vi "延迟测量.vi"() -> ()   [LabVIEW 2017]
uses:
  <vilib>/Utility/file.llb/Write Delimited Spreadsheet (string).vi
panel:
  in  "step":dbl=125.0 format="%#_13g"
  out "mean[ps]":dbl=-3.0179300175540487 format="%0.2f"
  out "standard output":string="CRITICAL WARNING: [Common 17-183] Failed to open handle vivado.jou. Please check access permission of directory 'C:\\Windows\\System32'. You should restart the application from a writable working directory.\r\nCRITICAL WARNING: [Common 17-183] Failed to open handle vivado.log. Please check access permission of directory 'C:\\Windows\\System32'. You should restart the application from a writable working directory.\r\n\r\n****** Vivado v2024.1 (64-bit)\r\n  **** SW Build 5076996 on Wed May 22 18:37:14 MDT 2024\r\n  **** IP Build 5075265 on Wed May 22 21:45:21 MDT 2024\r\n  **** SharedData Build 5076995 on Wed May 22 18:29:18 MDT 2024\r\n  **** Start of session at: Sat Mar  1 13:04:09 2025\r\n    ** Copyright 1986-2022 Xilinx, Inc. All Rights Reserved.\r\n    ** Copyright 2022-2024 Advanced Micro Devices, Inc. All Rights Reserved.\r\n\r\nsource {G:\\tdc\\2017\\program_fpga.tcl}\r\n# set_part {xc7k410tffg900-3}    \r\nINFO: [Coretcl 2-1500] The part has been set to 'xc7k410tffg900-3' for the current project only. Run set_part -help for more details. To evaluate different speed grades in the current design, use the set_speed_grade command, or use the open_checkpoint -part command to change the part used by an existing checkpoint design.\r\nset_part: Time (s): cpu = 00:00:06 ; elapsed = 00:00:07 . Memory (MB): peak = 617.039 ; gain = 204.969\r\n# open_hw_manager\r\n# connect_hw_server -allow_non_jtag              \r\nINFO: [Labtools 27-2285] Connecting to hw_server url TCP:localhost:3121\r\nINFO: [Labtools 27-3415] Connecting to cs_server url TCP:localhost:0\r\nINFO: [Labtools 27-3417] Launching cs_server...\r\nINFO: [Labtools 27-2221] Launch Output:\r\n\r\n\r\n******** Xilinx cs_server v2024.1.0\r\n  ****** Build date   : Mar 09 2024-08:00:37\r\n    **** Build number : 2024.1.1709942437\r\n      ** Copyright 2017-2022 Xilinx, Inc. All Rights Reserved.\r\n      ** Copyright 2022-2025 Advanced Micro Devices, Inc. All Rights Reserved.\r\n\r\n\r\n\r\n# open_hw_target {localhost:3121/xilinx_tcf/Xilinx/0000177f546201}\r\nINFO: [Labtoolstcl 44-466] Opening hw_target localhost:3121/xilinx_tcf/Xilinx/0000177f546201\r\n# set_property PROBES.FILE {} [get_hw_devices xc7k410t_0]\r\n# set_property FULL_PROBES.FILE {} [get_hw_devices xc7k410t_0]\r\n# set_property PROGRAM.FILE {G:/fpga_tdc/FPGA/muon_TDC/top_v120_v2.bit} [get_hw_devices xc7k410t_0]\r\n# program_hw_devices [get_hw_devices xc7k410t_0]\r\nINFO: [Labtools 27-3164] End of startup status: HIGH\r\nprogram_hw_devices: Time (s): cpu = 00:00:32 ; elapsed = 00:00:33 . Memory (MB): peak = 620.281 ; gain = 0.000\r\n# close_hw_target {localhost:3121/xilinx_tcf/Xilinx/0000177f546201}\r\nINFO: [Labtoolstcl 44-464] Closing hw_target localhost:3121/xilinx_tcf/Xilinx/0000177f546201\r\n# close_hw_manager\r\n# exit\r\nINFO: [Common 17-206] Exiting Vivado at Sat Mar  1 13:04:55 2025...\r\n"
  out "error out":errorcluster
  out "ping":bool=TRUE
  out "result":string[][](array[string])=[["_20250301_010502", "42", "-1963", "31", "16"], ["_20250301_010903", "42", "-3", "28", "0"]]
  in  "data  path":path=path "G:/tdc/2017/delay.csv"
  in  "stop":bool
  in  "PMT通道B":i32=42
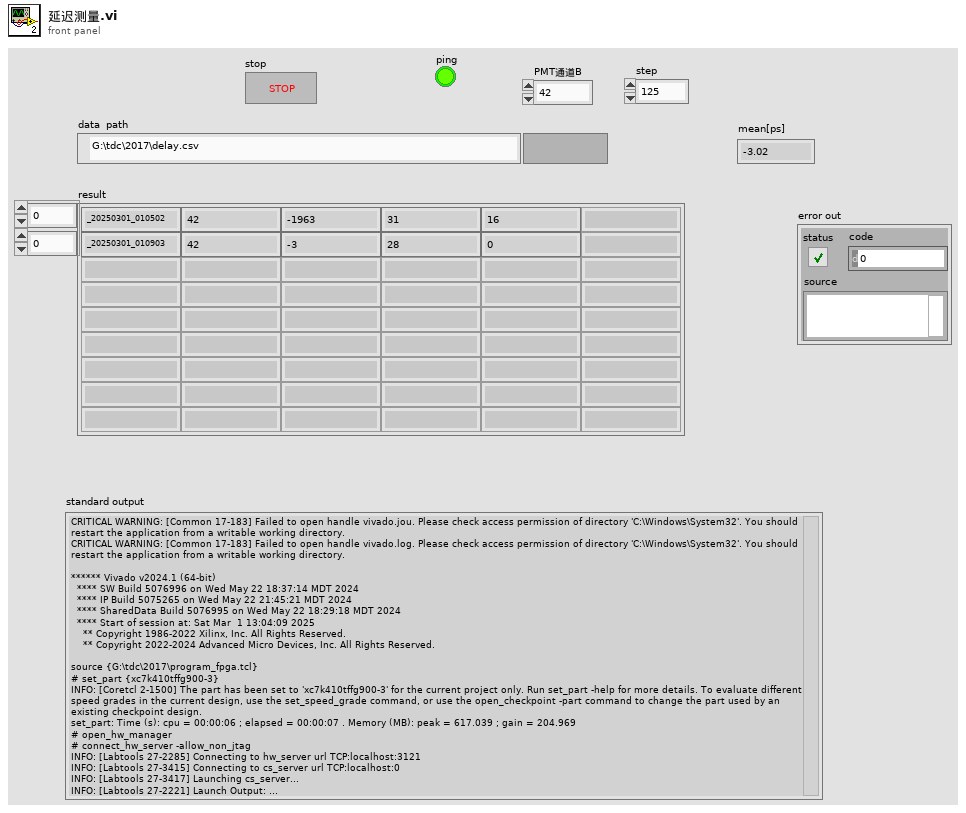
[diagram p1: front panel]
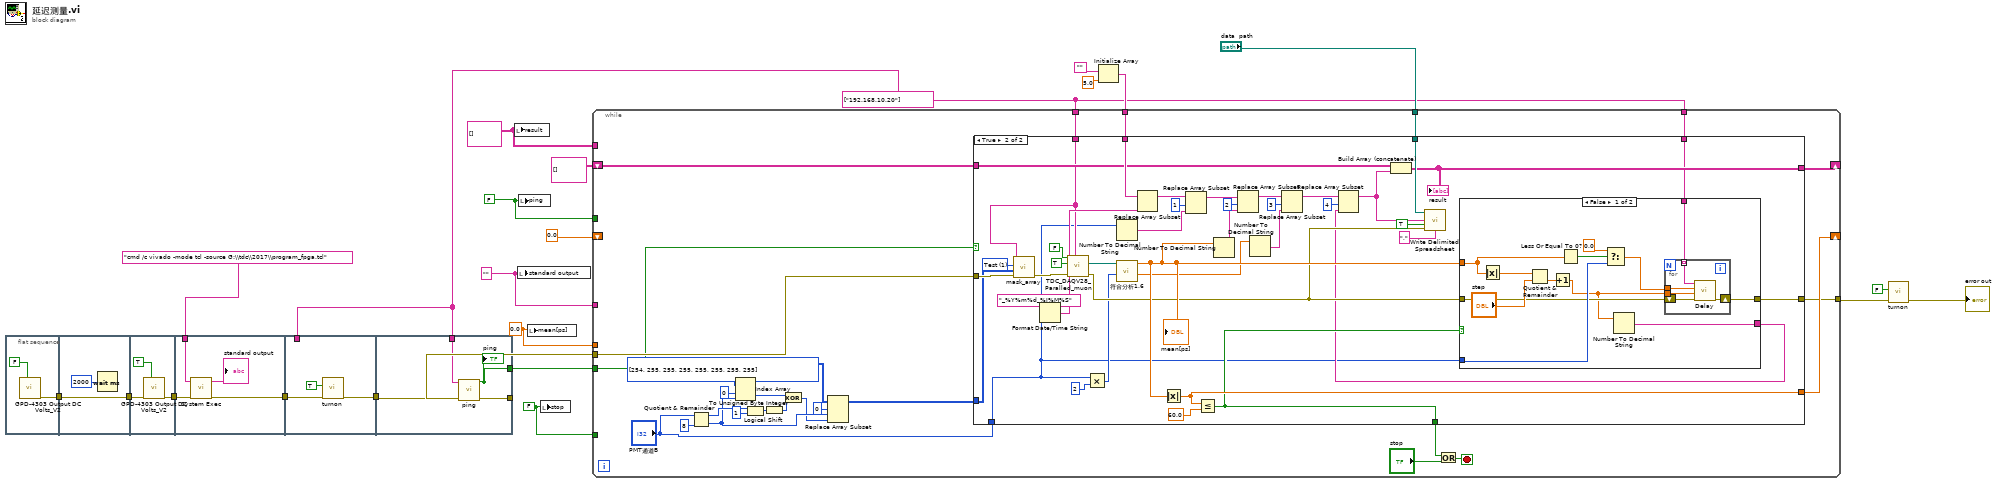
[diagram p0: block diagram]
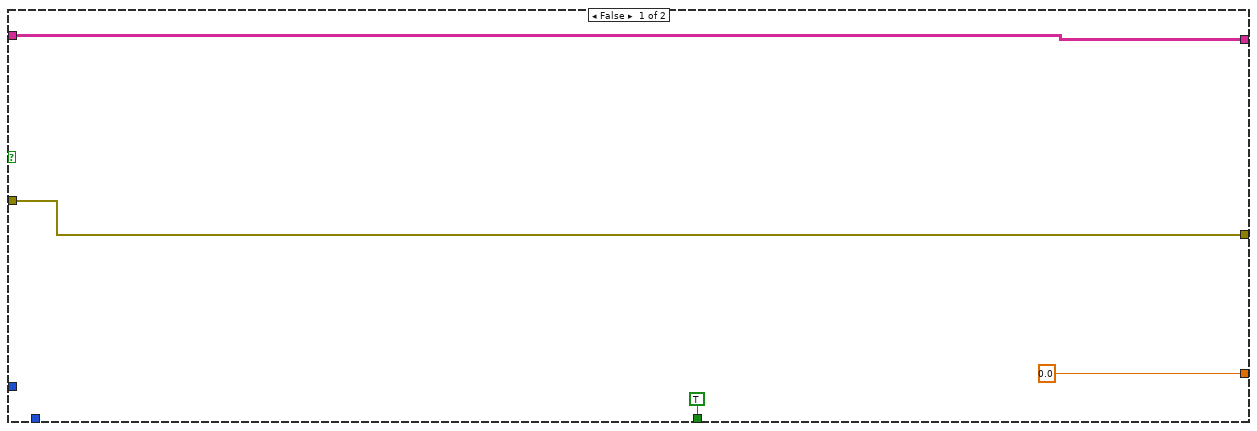
[diagram p2: hidden frame]
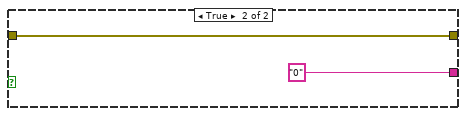
[diagram p3: hidden frame]
diagram:
  w7 = FALSE ("stop")
  w8 = 0.0 ("mean[ps]")
  w15 = "" ("standard output")
  w16 = FALSE ("ping")
  w17 = string[][] [] ("result")
  w4 = string[] ["192.168.10.20"] ("address")
  n1 = flat-sequence {
    tunnel: [w25] -> w14
    tunnel: w14 -> [w27]
    tunnel: [w27] -> w13
    tunnel: w13 -> [w29]
    tunnel: [w28] -> w12
    tunnel: w12 -> [w33]
    tunnel: "cmd /c vivado -mode tcl -source G:\\tdc\\2017\\program_fpga.tcl" ("command line") -> [w32]
    tunnel: [w34] -> w6
    tunnel: w6 -> [w37]
    tunnel: [w36] -> w5
    tunnel: w4 -> [_]
    tunnel: w5 -> [w41]
    tunnel: w4 -> [w40]
    tunnel: [w39] -> w11
    tunnel: [w38] -> w10
    frame #0 {
      n2 = call "GPD-4303 Output DC Volts_V2.vi"("Enable Output (T: Enable)"=FALSE) -> ("error out"=w25:errorcluster)  [unwired: 8 in, 2 out]
    }
    frame #1 {
      n3 = Wait (ms)(milliseconds to wait=u32 2000) -> ()  [unwired: 1 out]
    }
    frame #2 {
      n4 = call "GPD-4303 Output DC Volts_V2.vi"("Enable Output (T: Enable)"=TRUE, "error in (no error)"=w29) -> ("error out"=w28:errorcluster)  [unwired: 7 in, 2 out]
    }
    frame #3 {
      n5 = call <vilib>:"System Exec.vi"("error in (no error)"=w33, "command line"=w32) -> ("error out"=w34:errorcluster, "standard output"=→"standard output":string)  [unwired: 6 in, 2 out]
    }
    frame #4 {
      n6 = call "turnon.vi"("error in (no error)"=w37, "Enable Output (T: Enable)"=TRUE) -> ("error out"=w36:errorcluster)  [unwired: 9 in]
    }
    frame #5 {
      n7 = call "ping.vi"("error in (no error)"=w41, "address"=w40) -> ("error out"=w39:errorcluster, "ping"=w38:bool)  [unwired: 7 in, 1 out]
      "ping" <- w38
    }
  }
  n8 = local write "result"(w17) -> ()
  n9 = local write "standard output"(w15) -> ()
  n10 = local write "ping"(w16) -> ()
  n11 = local write "mean[ps]"(w8) -> ()
  n12 = local write "stop"(w7) -> ()
  n13 = Initialize Array("", 5.0 ("element")) -> (w19:string[])
  n14 = while {
    tunnel: w4 -> [w47]
    shift-right: [w65] -> _
    shift-left: 0.0 ("t") -> [_]
    tunnel: "data  path" -> [w63]
    tunnel: w19 -> [w62]
    shift-right: [w61] -> _
    shift-left: string[][] [] -> [w60]
    tunnel: [w46] -> w2
    tunnel: w17 -> [_]
    tunnel: w16 -> [_]
    tunnel: w15 -> [_]
    tunnel: w4 -> [w45]
    tunnel: w11 -> [w44]
    tunnel: w10 -> [w43]
    tunnel: w8 -> [_]
    tunnel: w7 -> [_]
    stop <- w67 stop-if-true
    w55 = u8[][] [[254, 255, 255, 255, 255, 255, 255, 255]] ("Test")
    n15 = Quotient & Remainder(x="PMT通道B", y=8) -> (x-y*floor(x/y)=w56:i32, floor(x/y)=w54:i32)
    n16 = Index Array(array=w55, index (row)=0 ("disabled index (row)"), index (col)=w54) -> (element=w52:u8)
    n17 = Logical Shift(y=w56, x=u32 1) -> (x << y=w50:u32)
    n18 = To Unsigned Byte Integer(number=w50) -> (unsigned 8bit integer=w49:u8)
    n19 = Exclusive Or(1:w49, 2:w52) -> (0:w51:u8)
    n20 = Replace Array Subset(array=w55, new element=w51, index (row)=0, index (col)=w54) -> (w48:u8[][])
    n21 = case shown="True" w43 {
      tunnel: [0.0 w107] -> w65
      tunnel: [TRUE w106] -> w64
      tunnel: w63 -> [_ w103]
      tunnel: w62 -> [_ w102]
      tunnel: [w71 w88] -> w61
      tunnel: w60 -> [w71 w87]
      tunnel: w44 -> [w70 w80]
      tunnel: w48 -> [_ w79]
      tunnel: w47 -> [_ w78]
      tunnel: [w70 w76] -> w46
      tunnel: w45 -> [_ w75]
      tunnel: "PMT通道B" -> [_ w72]
      frame False {
      }
      frame True {
        w77 = u16 1 items=["default", "Test", "NormalUse"] ("下拉列表")
        n22 = call "mask_array.vi"("error in (no error)"=w80, "Test"=w79, "下拉列表"=w77, "address"=w78) -> ("error out"=w81:errorcluster)  [unwired: 7 in]
        n23 = Format Date/Time String(time format string (%c)="_%Y%m%d_%I%M%S") -> (date/time string=w100:string)  [unwired: 2 in]
        n24 = call "TDC_DAQV28_Paralled_muon.vi"("address"=w78, "error in (no error)"=w81, "save data"=TRUE, "SMA mode"=FALSE) -> ("error out 3"=w83:errorcluster, "csv path"=w109:path)  [unwired: 5 in, 1 out]
        n25 = Multiply(x=w72, y=2) -> (x*y=w73:i32)
        n26 = Number To Decimal String(number=w72) -> (decimal integer string=w97:string)  [unwired: 1 in]
        n27 = call "符合分析1.6.vi"("通道B"=w73, "file path (dialog if empty)"=w109) -> ("Fitting Sigma"=w90:dbl, "mean[ps]"=w93:dbl)  [unwired: 5 in, 3 out]
        "mean[ps]" <- w93
        n28 = Replace Array Subset(array=w102, new element=w100) -> (w99:string[])  [unwired: 1 in]
        n29 = Absolute Value(x=w93) -> (abs(x)=w107:dbl)
        n30 = Replace Array Subset(array=w99, new element=w97, index=1) -> (w96:string[])
        n31 = Less Or Equal?(x=w107, y=60.0) -> (x <= y?=w106:bool)
        n32 = Number To Decimal String(number=w93) -> (decimal integer string=w94:string)  [unwired: 1 in]
        n33 = Replace Array Subset(array=w96, new element=w94, index=2) -> (w92:string[])
        n34 = Number To Decimal String(number=w90) -> (decimal integer string=w89:string)  [unwired: 1 in]
        n35 = Replace Array Subset(array=w92, new element=w89, index=3) -> (w86:string[])
        n36 = case shown="False" w106 {
          tunnel: w93 -> [w122 _]
          tunnel: w72 -> [w120 _]
          tunnel: w83 -> [w118 w130]
          tunnel: [w116 "0"] -> w82
          tunnel: [w115 w130] -> w76
          tunnel: w75 -> [w113 _]
          frame False {
            n37 = Absolute Value(x=w122) -> (abs(x)=w124:dbl)
            n38 = Quotient & Remainder(x=w124, y="step") -> (floor(x/y)=w117:dbl)  [unwired: 1 out]
            n39 = Increment(x=w117) -> (x+1=w112:dbl)
            n40 = Less Or Equal To 0?(x=w122) -> (x <= 0?=w114:bool)
            n41 = Select(t=0.0, s=w114, f=w120) -> (s? t:f=w119:dbl)
            n42 = Number To Decimal String(number=w112) -> (decimal integer string=w116:string)  [unwired: 1 in]
            n43 = for {
              tunnel: w119 -> [w129]
              tunnel: w112 -> [w127]
              shift-right: [w126] -> w115
              shift-left: w118 -> [w128]
              tunnel: w113 -> [w125] mode=indexing
              n44 = call "Delay.vi"("error in (no error)"=w128, "delay_value"=w127, "channel"=w129, "IP address"=w125) -> ("error out"=w126:errorcluster)  [unwired: 7 in]
            }
          }
          frame True {
          }
        }
        n45 = Replace Array Subset(array=w86, new element=w82, index=4) -> (w85:string[])
        n46 = Build Array (concatenate)(w87, w85) -> (w88:string[][])
        "result" <- w88
        n47 = call-poly <vilib>:"Write Delimited Spreadsheet.vi"("file path (dialog if empty)"=w103, "1D data"=w85, "append to file? (new file:F)"=TRUE, "error in (no error)"=w83, "delimiter (\\t)"="," ("delimiter (\\t)")) -> ()  [unwired: 9 in, 2 out]
      }
    }
    n48 = Or(x=w64, y="stop") -> (x .or. y?=w67:bool)
  }
  n49 = call "turnon.vi"("error in (no error)"=w2, "Enable Output (T: Enable)"=FALSE) -> ("error out"=→"error out":errorcluster)  [unwired: 9 in]
